vi "Destroy.vi"(8 "error in (no error)":errorcluster, 11 "Game in":refnum<class "Game.lvclass">) -> (0 "error out":errorcluster, 3 "FPGA_ref":T1)   [LabVIEW 2019, in "RT_Game.lvlib" / "Game.lvclass"]
uses:
  Game.lvclass
  FPGA_Interface.ctl
  Game.lvclass/Game.ctl
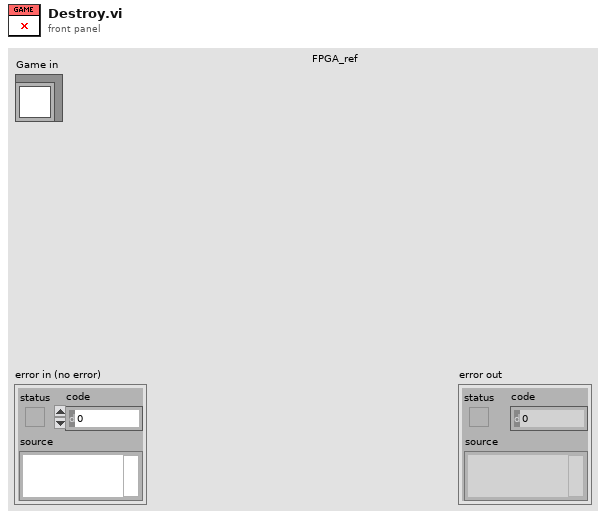
[diagram p1: front panel]
types:
  T1 = typedef "FPGA_Interface.ctl" = refnum<k20>
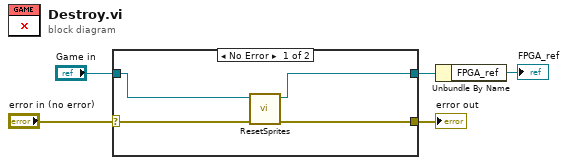
[diagram p0: block diagram]
diagram:
  n1 = case shown="No Error" "error in (no error)" {
    selector: "error in (no error)" -> [w9 w11]
    tunnel: [w8 w11] -> w4
    tunnel: [w6 w10] -> w2
    tunnel: "Game in" -> [w7 w10]
    frame No Error {
      n2 = call "ResetSprites.vi"("error in (no error)"=w9, "Game in"=w7) -> ("error out"=w8:errorcluster, "Game out"=w6:refnum<class "Game.lvclass">)  [unwired: 8 in]
    }
    frame Error {
    }
  }
  "error out" <- w4
  n3 = Unbundle By Name(w2) -> ("FPGA_ref"=→"FPGA_ref":T1)
